vi "Window-ROI Grouping.vi"() -> ()   [LabVIEW 2013]
uses:
  Typedefs/ROI grp-window ctrl refs.ctl
  Typedefs/ROI grp-Internal register.ctl
  ROI Selection Interface/ROI group info cluster.ctl
  Typedefs/Group sel cluster.ctl
  Globals/gl_ROI grp window globals.vi
  Global Variables/General Globals.vi
  Global variables/gl_Functional Imaging-Global variables.vi
panel:
  in  "Table":string[][](table) caption="#\n\n\nROI Groups Table"
  in  "Cancel":bool
  in  "Save":bool
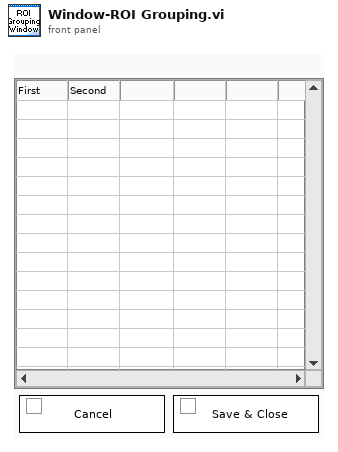
[diagram p1: front panel]
types:
  T1 = typedef "ROI grp-window ctrl refs.ctl" = cluster{"This VI":refnum<vi>, "Pane":refnum<vi>, "Table":refnum<vi>}
  T2 = enum8{"Enabled", "Disabled", "Disabled and Grayed Out"}
  T3 = typedef "ROI grp-Internal register.ctl" = cluster{"ROI groups header file data":string[][], "Groups setup out":T4[], "[Groups]":T6[]}
  T4 = typedef "ROI group info cluster.ctl" = cluster{"Group name":string, "# ROI in group":i32, "ROI numbers in group":i32[], "Group region specifier cluster":T5}
  T5 = typedef "ROI Descriptor" = cluster{"Global Rectangle":i32[], "Contours":cluster{"ID":enum32{"External", "Internal"}, "Type":u32, "Coordinates":i32[]}[]}
  T6 = typedef "Group sel cluster.ctl" = cluster{"Group number":string, "Group Name":string, "Visibility":bool, "Highlight":bool}
  T7 = typedef "LVPoint32TypeDef.ctl" = cluster{"Horizontal":i32, "Vertical":i32}
  T8 = typedef "LVRowAndColumnTypeDef.ctl" = cluster{"Row":i32, "Column":i32}
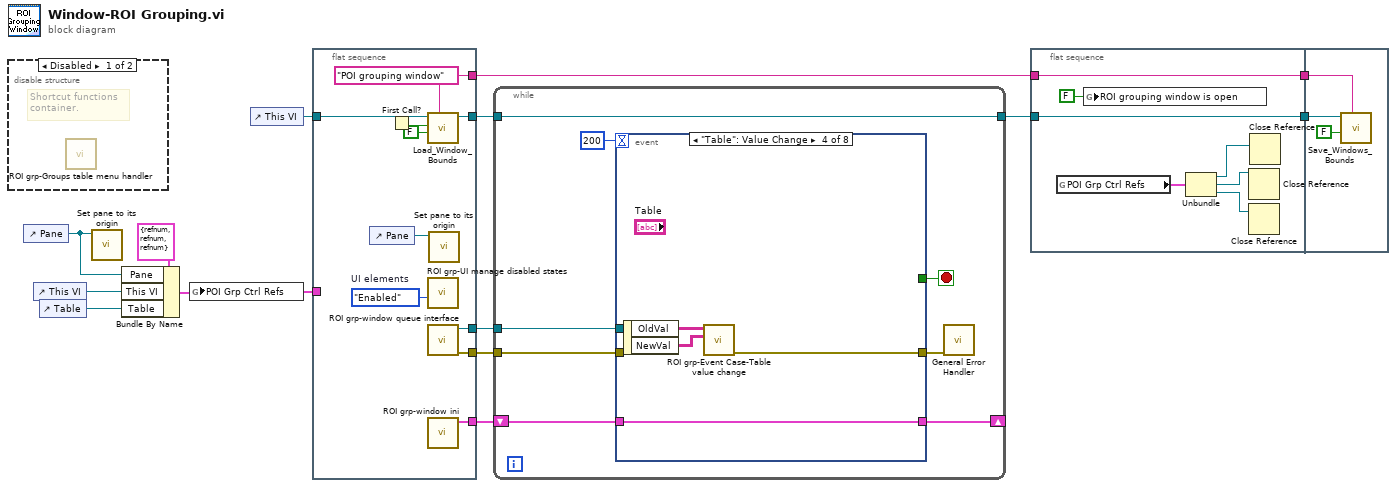
[diagram p0: block diagram]
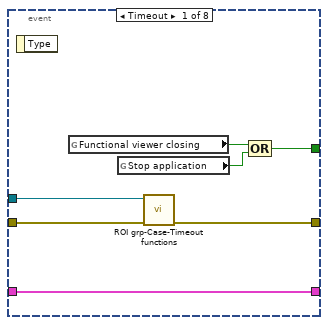
[diagram p3: hidden frame]
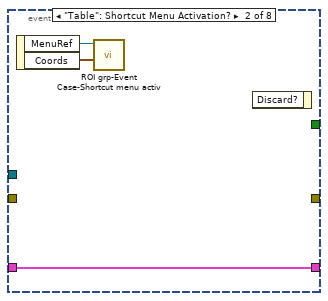
[diagram p4: hidden frame]
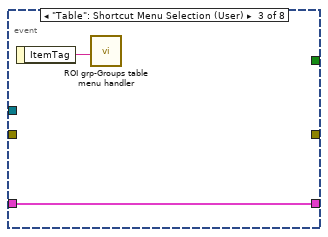
[diagram p5: hidden frame]
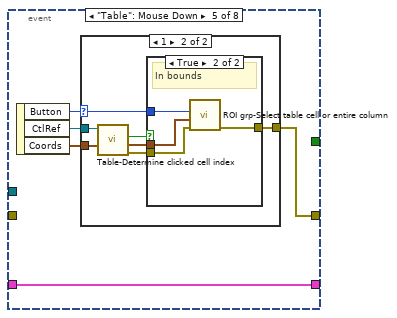
[diagram p6: hidden frame]
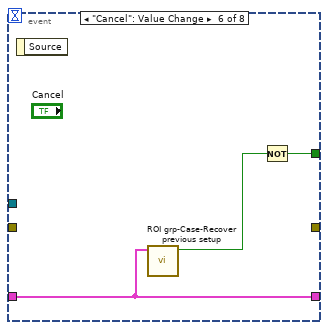
[diagram p9: hidden frame]
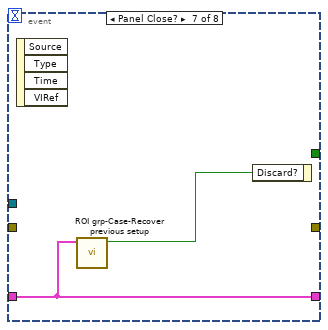
[diagram p10: hidden frame]
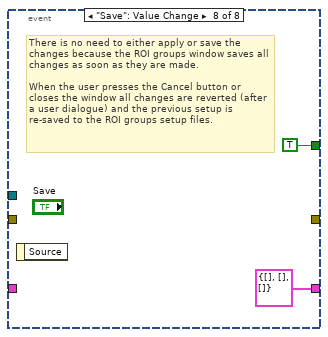
[diagram p11: hidden frame]
diagram:
  n1 = disable-structure shown="Disabled" {
    frame Disabled {
      # "Shortcut functions\ncontainer."
      n2 = call "ROI grp-Groups table menu handler.vi"() -> ()  [unwired: 12 in]
    }
    frame Enabled {
    }
  }
  n3 = control-ref of="Pane"() -> (w8:refnum<vi>)
  n4 = control-ref of="This VI"() -> (w10:refnum<vi>)
  n5 = control-ref of="Table"() -> (w11:refnum<vi>)
  n6 = call "Set pane to its origin.vi"("Pane Reference"=w8) -> ()  [unwired: 9 in, 2 out]
  n7 = Bundle By Name(cluster=T1 {"This VI"=refnum, "Pane"=refnum, "Table"=refnum} ("output cluster"), "Pane"=w8, "This VI"=w10, "Table"=w11) -> (w9:T1)
  n8 = global write "gl_ROI grp window globals.vi" "POI Grp Ctrl Refs"(w9) -> ()
  n9 = control-ref of="This VI"() -> (w7:refnum<vi>)
  n10 = flat-sequence {
    tunnel: [w23] -> w14
    tunnel: [w22] -> w13
    tunnel: [w21] -> w12
    tunnel: w9 -> [_]
    tunnel: w7 -> [w20]
    tunnel: [w19] -> w6
    tunnel: [w18] -> w4
    frame #0 {
      w18 = "POI grouping window" ("Window Name (i.e. Key)")
      w24 = T2."Enabled"  # UI elements
      n11 = control-ref of="Pane"() -> (w15:refnum<vi>)
      n12 = First Call?() -> (First Call?: T/F=w16:bool)
      n13 = call "Load_Window_Bounds.vi"("Window Name (i.e. Key)"=w18, "Disable"=FALSE, "First Call"=w16, "Window VI's Ref"=w20) -> ("reference out"=w19:refnum<vi>)  [unwired: 4 in, 3 out]
      n14 = call "ROI grp-UI manage disabled states.vi"("UI elemente enabled?"=w24) -> ()  [unwired: 10 in, 1 out]
      n15 = call "ROI grp-window queue interface.vi"() -> ("error out"=w22:errorcluster, "ROI grouping window queue"=w23:refnum<queue>)  [unwired: 10 in]
      n16 = call "ROI grp-window ini.vi"() -> ("ROI groups new setup"=w21:T3)  [unwired: 10 in, 1 out]
      n17 = call "Set pane to its origin.vi"("Pane Reference"=w15) -> ()  [unwired: 9 in, 2 out]
    }
  }
  n18 = while {
    tunnel: w14 -> [w30]
    tunnel: w13 -> [w29]
    tunnel: [w26] -> w5
    tunnel: w6 -> [w26]
    shift-right: [w25] -> _
    shift-left: w12 -> [w28]
    stop <- w31 stop-if-true
    n19 = event shown="[3] \"Table\": Value Change" {
      selector: _ -> [_ _ _ _ _ _ _ _]
      dyn-events: _ -> [_ _ _ _ _ _ _ _]
      timeout: 200 -> [_ _ _ _ _ _ _ _]
      tunnel: [w34 _ _ _ _ w66 _ TRUE] -> w31
      tunnel: w30 -> [w39 _ _ _ _ _ _ _]
      tunnel: w29 -> [w38 _ _ _ _ _ _ _]
      tunnel: w28 -> [w33 w42 w43 w45 w50 w68 w70 _]
      tunnel: [w37 _ _ w46 w51 _ _ _] -> w27
      tunnel: [w33 w42 w43 w45 w50 w68 w70 T3 {"ROI groups header file data"=[], "Groups setup out"=[], "[Groups]"=[]} ("ROI groups new setup")] -> w25
      event Timeout {
        n20 = event-data() -> ()  [unwired: 1 in, 1 out]
        n21 = global read "gl_Functional Imaging-Global variables.vi" "Functional viewer closing"() -> (w36:bool)
        n22 = global read "General Globals.vi" "Stop application"() -> (w35:bool)
        n23 = call "ROI grp-Case-Timeout functions.vi"("error in (no error)"=w38, "ROI grouping window queue"=w39) -> ("error out"=w37:errorcluster)  [unwired: 9 in]
        n24 = Compound Arithmetic op=OR(w36, w35) -> (w34:bool)
      }
      event "Table": Shortcut Menu Activation? {
        n25 = event-data() -> ("MenuRef"=w41:refnum<k9>, "Coords"=w40:T7)  [unwired: 1 in]
        n26 = call "ROI grp-Event Case-Shortcut menu activ.vi"("Coords"=w40, "[Groups] menu ref"=w41) -> ()  [unwired: 9 in, 1 out]
        n27 = event-data() -> ()  [unwired: 2 in, 1 out]
      }
      event "Table": Shortcut Menu Selection (User) {
        n28 = event-data() -> ("ItemTag"=w44:string)  [unwired: 1 in]
        n29 = call "ROI grp-Groups table menu handler.vi"("ItemTag"=w44) -> ()  [unwired: 11 in]
      }
      event "Table": Value Change {
        n30 = event-data() -> ("OldVal"=w47:string[][], "NewVal"=w48:string[][])  [unwired: 1 in]
        n31 = call "ROI grp-Event Case-Table value change.vi"("NewVal"=w48, "OldVal"=w47) -> ("error out"=w46:errorcluster)  [unwired: 9 in]
      }
      event "Table": Mouse Down {
        n32 = event-data() -> ("Button"=w49:u16, "CtlRef"=w53:refnum<vi>, "Coords"=w52:T7)  [unwired: 1 in]
        n33 = case shown="1" w49 {
          selector: w49 -> [_ w54]
          tunnel: w53 -> [_ w60]
          tunnel: w52 -> [_ w59]
          tunnel: [_ w55] -> w51
          frame Default {
          }
          frame 1 {
            n34 = call "Table-Determine clicked cell index.vi"("Coords"=w59, "Table in"=w60) -> ("error out"=w56:errorcluster, "Cell Position"=w58:T8, "In Bounds?"=w57:bool)  [unwired: 6 in, 1 out]
            n35 = case shown="True" w57 {
              tunnel: w54 -> [_ w65]
              tunnel: w58 -> [_ w64]
              tunnel: w56 -> [w61 w63]
              tunnel: [w61 w62] -> w55
              frame False {
              }
              frame True {
                # "In bounds"
                n36 = call "ROI grp-Select table cell or entire column.vi"("error in (no error)"=w63, "Cell Position"=w64, "Button (1=left 2=right)"=w65) -> ("error out"=w62:errorcluster)  [unwired: 8 in]
              }
            }
          }
        }
      }
      event "Cancel": Value Change {
        n37 = event-data() -> ()  [unwired: 1 in, 1 out]
        n38 = call "ROI grp-Case-Recover previous setup.vi"("POI groups initial setup"=w68) -> ("Window close was cancelled"=w67:bool)  [unwired: 9 in, 1 out]
        n39 = Not(x=w67) -> (.not. x?=w66:bool)
      }
      event Panel Close? {
        n40 = event-data() -> ()  [unwired: 1 in, 4 out]
        n41 = call "ROI grp-Case-Recover previous setup.vi"("POI groups initial setup"=w70) -> ("Window close was cancelled"=w69:bool)  [unwired: 9 in, 1 out]
        n42 = event-data("Discard?"=w69) -> ()  [unwired: 1 in, 1 out]
      }
      event "Save": Value Change {
        # "There is no need to either apply or save the changes because the ROI groups window saves all changes as soon as they are made.\n\nWhen the user presses the Cancel button or closes the window all changes are reverted (after a user dialogue) and the previous setup is re-saved to the ROI groups setup files."
        n43 = event-data() -> ()  [unwired: 1 in, 1 out]
      }
    }
    n44 = call <vilib>:"General Error Handler.vi"("error in (no error)"=w27) -> ()  [unwired: 10 in, 5 out]
  }
  n45 = flat-sequence {
    tunnel: w4 -> [w78]
    tunnel: w5 -> [w79]
    tunnel: [w79] -> w2
    tunnel: [w78] -> w1
    tunnel: w2 -> [w82]
    tunnel: w1 -> [w80]
    frame #0 {
      n46 = global read "gl_ROI grp window globals.vi" "POI Grp Ctrl Refs"() -> (w76:T1)
      n47 = global write "gl_ROI grp window globals.vi" "ROI grouping window is open"(FALSE ("POI grouping window is open")) -> ()
      n48 = Unbundle(w76) -> ("This VI"=w75:refnum<vi>, "Pane"=w74:refnum<vi>, "Table"=w73:refnum<vi>)
      n49 = Close Reference(reference=w74) -> ()  [unwired: 1 in, 1 out]
      n50 = Close Reference(reference=w73) -> ()  [unwired: 1 in, 1 out]
      n51 = Close Reference(reference=w75) -> ()  [unwired: 1 in, 1 out]
    }
    frame #1 {
      n52 = call "Save_Windows_Bounds.vi"("Window Name (i.e. Key)"=w80, "Front Panel Window:Open"=FALSE, "Window VI's Ref"=w82) -> ()  [unwired: 8 in, 1 out]
    }
  }
